vi "TestThor.vi"() -> ()   [LabVIEW 2019, in "TEMPerHUM.lvlib"]
uses:
  TEMPerHUM.lvlib
panel:
  out "error out":errorcluster
  out "TH1 Value":dbl caption="Temperature Value"
  out "Humidity":dbl
  out "Temperature":dbl
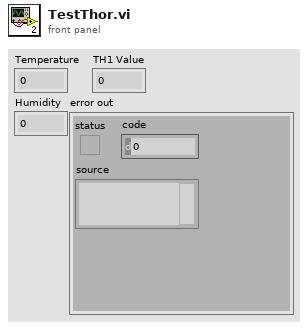
[diagram p1: front panel]
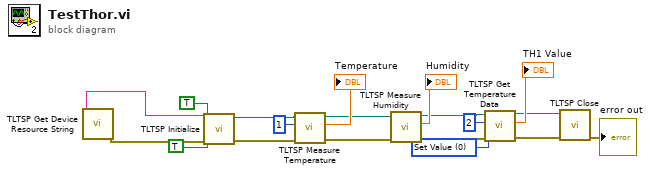
[diagram p0: block diagram]
diagram:
  w13 = i16 0 items=["Set Value", "Minimum value", "Maximum value"] ("Attribute (Set Value)")
  n1 = call "TLTSP Get Device Resource String.vi"() -> ("error out"=w6:errorcluster, "Resource Name"=w7:string)  [unwired: 9 in, 1 out]
  n2 = call "TLTSP Initialize.vi"("error in (no error)"=w6, "Reset Device (Reset Device)"=TRUE, "ID Query (Do Query)"=TRUE, "resource name"=w7) -> ("error out"=w5:errorcluster, "instrument handle out"=w8:refnum<visa-resource-name>)  [unwired: 6 in]
  n3 = call "TLTSP Measure Temperature.vi"("error in (no error)"=w5, "Channel (1)"=u16 1, "instrument handle"=w8) -> ("error out"=w4:errorcluster, "Temperature"=→"Temperature":dbl, "instrument handle out"=w18:refnum<visa-resource-name>)  [unwired: 6 in]
  n4 = call "TLTSP Measure Humidity.vi"("error in (no error)"=w4, "instrument handle"=w18) -> ("error out"=w3:errorcluster, "Humidity"=→"Humidity":dbl, "instrument handle out"=w15:refnum<visa-resource-name>)  [unwired: 7 in]
  n5 = call <instrlib>:"TLTSP Get Temperature Data.vi"("error in (no error)"=w3, "Attribute (Set Value)"=w13, "Channel (1)"=u16 2, "instrument handle"=w15) -> ("error out"=w2:errorcluster, "Temperature Value"=→"TH1 Value":dbl, "instrument handle out"=w11:refnum<visa-resource-name>)  [unwired: 5 in]
  n6 = call "TLTSP Close.vi"("error in (no error)"=w2, "instrument handle"=w11) -> ("error out"=→"error out":errorcluster)  [unwired: 9 in]
